vi "GOOP_CheckForUMLModeller.vi"() -> (2 "UML-Modeller VI Path":path, 3 "UML Modeller Exists":bool)   [LabVIEW 2020]
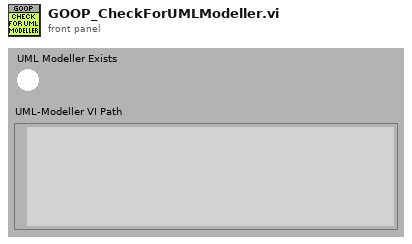
[diagram p1: front panel]
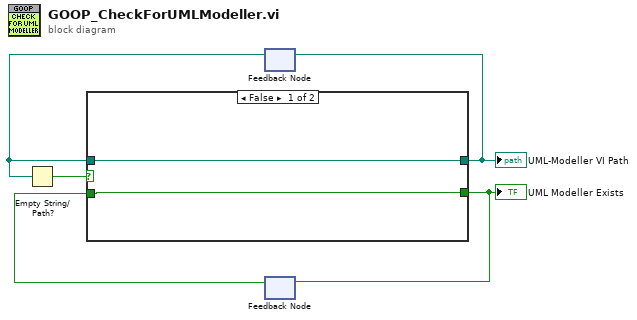
[diagram p0: block diagram]
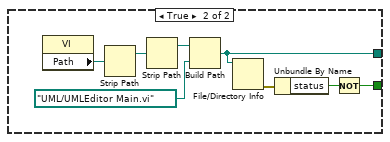
[diagram p2: hidden frame]
diagram:
  n1 = feedback #1() -> (w1:path)  [unwired: 1 in]
  n2 = Empty String/Path?(string/path=w1) -> (empty?=w3:bool)
  n3 = feedback #2() -> (w2:bool)  [unwired: 1 in]
  n4 = case shown="False" w3 {
    tunnel: [w6 w9] -> w5
    tunnel: [w7 w8] -> w4
    tunnel: w2 -> [w6 _]
    tunnel: w1 -> [w7 _]
    frame False {
    }
    frame True {
      n5 = property class="VI"() -> ("Path"=w15:path)  [unwired: 2 in, 2 out]
      n6 = Strip Path(path=w15) -> (stripped path=w14:path)  [unwired: 1 out]
      n7 = Strip Path(path=w14) -> (stripped path=w13:path)  [unwired: 1 out]
      n8 = Build Path(base path=w13, name or relative path=path "UML/UMLEditor Main.vi") -> (appended path=w8:path)
      n9 = File/Directory Info(path=w8) -> (error out=w10:errorcluster)  [unwired: 1 in, 6 out]
      n10 = Unbundle By Name(w10) -> ("status"=w11:bool)
      n11 = Not(x=w11) -> (.not. x?=w9:bool)
    }
  }
  "UML-Modeller VI Path" <- w4
  "UML Modeller Exists" <- w5
  n12 = feedback-in #1(w4) -> ()
  n13 = feedback-in #2(w5) -> ()
